vi "Set Output Pct.vi"(8 "error in (no error)":errorcluster, 10 "Output %":dbl, 11 "Pump in":refnum<class "Pump.lvclass">) -> (0 "error out":errorcluster, 3 "Pump out":refnum<class "Pump.lvclass">)   [LabVIEW 2014, in "Pump.lvclass"]
uses:
  Pump.lvclass
  Pump.lvclass/Pump.ctl
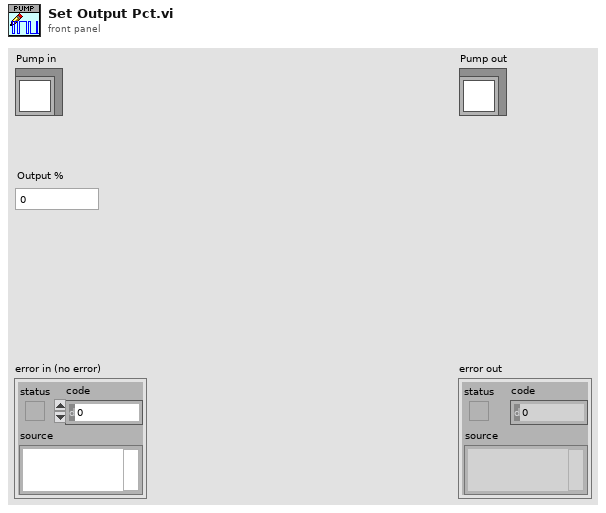
[diagram p1: front panel]
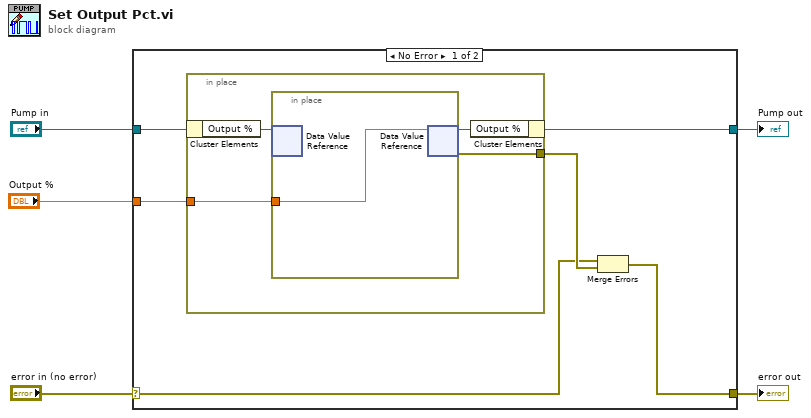
[diagram p0: block diagram]
diagram:
  n1 = case shown="No Error" "error in (no error)" {
    selector: "error in (no error)" -> [w7 w18]
    tunnel: [w6 w18] -> w4
    tunnel: [w9 w17] -> w2
    tunnel: "Pump in" -> [w11 w17]
    tunnel: "Output %" -> [w10 _]
    frame No Error {
      n2 = in-place {
        in-place-border: w10 -> [w14]
        in-place-border: [w12] -> w8
        n3 = in-place-cluster #1(w11) -> ("Output %"=w15:refnum<data-value>)
        n4 = in-place {
          in-place-border: w14 -> [w16]
          n5 = in-place-dvr #2(w15) -> ()  [unwired: 2 out]
          n6 = in-place-dvr #2(w16) -> (w13:refnum<data-value>, w12:errorcluster)
        }
        n7 = in-place-cluster #1("Output %"=w13) -> (w9:refnum<class "Pump.lvclass">)
      }
      n8 = Merge Errors(w7, w8) -> (w6:errorcluster)
    }
    frame Error {
    }
  }
  "error out" <- w4
  "Pump out" <- w2
